vi "setUp.vi"(8 "error in (no error)":errorcluster, 11 "reference in":refnum<class "TestMysqlDatabaseConfiguration.lvclass">) -> (0 "error out":errorcluster, 3 "reference out":refnum<class "TestMysqlDatabaseConfiguration.lvclass">)   [LabVIEW 2020, in "mysql tests.lvlib" / "TestMysqlDatabaseConfiguration.lvclass"]
doc: "setUp runs prior to the test method during test execution. Use this method to initialize any object data required by your tests."
uses:
  TestMysqlDatabaseConfiguration.lvclass
  C:/Program Files/National Instruments/LabVIEW 2020/vi.lib/addons/_JKI Toolkits/VI Tester/TestCase.llb/TestCase.lvclass
  TestMysqlDatabaseConfiguration.lvclass/TestMysqlDatabaseConfiguration.ctl
  externals/mysql/Source/mysql.net/mysql.lvclass
  D:/Project/Labview-Projects/database-configuration/externals/database-interface/IDatabase/IDatabase/IDatabase.lvclass
  <vilib>/addons/_JKI Toolkits/VI Tester/TestCase.llb/TestCase.lvclass
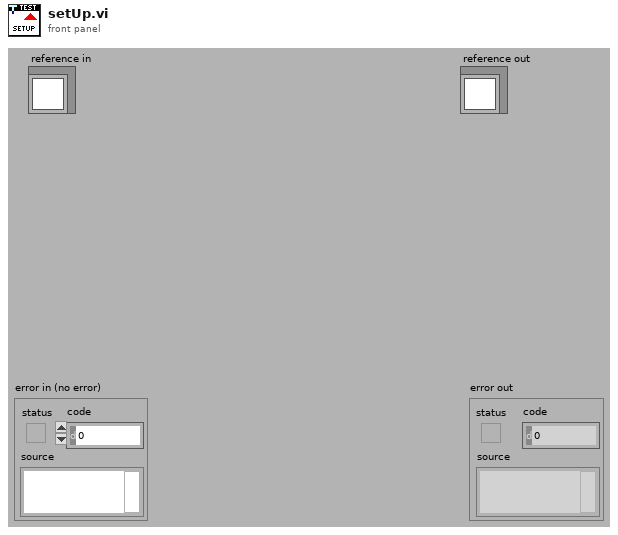
[diagram p1: front panel]
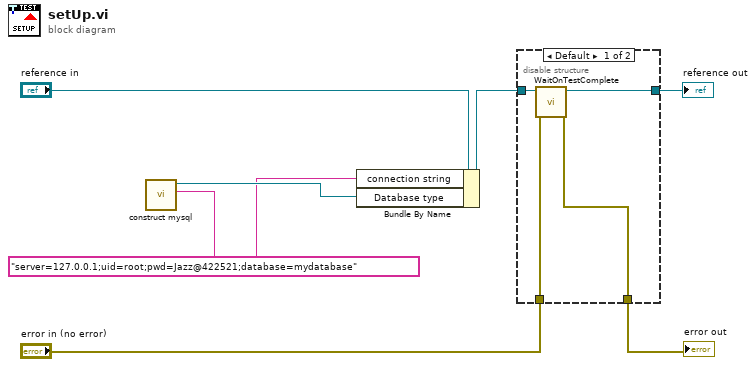
[diagram p0: block diagram]
diagram:
  w1 = "server=127.0.0.1;uid=root;pwd=Jazz@422521;database=mydatabase" ("Name")
  n1 = call "construct mysql.vi"("Connection string"=w1) -> ("mysql out"=w2:refnum<class "mysql.lvclass">)  [unwired: 9 in, 1 out]
  n2 = Bundle By Name(cluster="reference in", "connection string"=w1, "Database type"=w2) -> (w3:refnum<class "TestMysqlDatabaseConfiguration.lvclass">)
  n3 = disable-structure shown="Default" {
    disable-tunnel: "error in (no error)" -> [w11 w12]
    disable-tunnel: [w10 w12] -> w6
    disable-tunnel: [w9 w13] -> w4
    disable-tunnel: w3 -> [w8 w13]
    frame condition #0 (active) {
      n4 = call <vilib>:"WaitOnTestComplete.vi"("error in (no error)"=w11, "TestCase in"=w8) -> ("error out"=w10:errorcluster, "TestCase out"=w9:refnum<class "TestMysqlDatabaseConfiguration.lvclass">)  [unwired: 8 in]
    }
    frame condition #1 {
    }
  }
  "error out" <- w6
  "reference out" <- w4
